vi "Client Test.vi"() -> ()   [LabVIEW 2019, in "Simple_client.lvlib" / "Simple_client.lvclass"]
uses:
  Simple_client.lvclass
  RPC Messages/simpleMsgReq/simpleMsgReq_Data.ctl
  RPC Messages/simpleMgsReply/simpleMgsReply_Data.ctl
panel:
  out "Response Data":T1
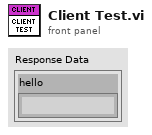
[diagram p1: front panel]
types:
  T1 = typedef "Simple_client.lvlib/Simple_client.lvclass/simpleMgsReply_Data.ctl" = cluster{"hello":string}
  T2 = typedef "Simple_client.lvlib/Simple_client.lvclass/simpleMsgReq_Data.ctl" = cluster{"name":string}
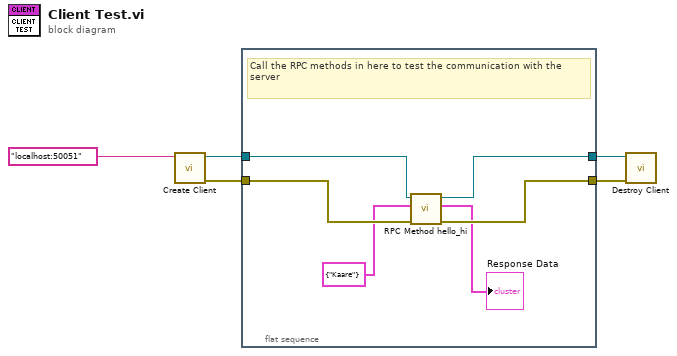
[diagram p0: block diagram]
diagram:
  n1 = call "Create Client.vi"("address"="localhost:50051") -> ("error out"=w1:errorcluster, "gRPC Client out"=w3:refnum<class "Simple_client.lvclass">)  [unwired: 9 in]
  n2 = flat-sequence {
    tunnel: [w10] -> w4
    tunnel: w3 -> [w11]
    tunnel: [w9] -> w2
    tunnel: w1 -> [w8]
    frame #0 {
      # "Call the RPC methods in here to test the communication with the server"
      n3 = call "RPC Method hello_hi.vi"("error in (no error)"=w8, "Request Data"=T2 {"name"="Kaare"}, "gRPC Client in"=w11) -> ("error out"=w9:errorcluster, "Response Data"=→"Response Data":T1, "gRPC Client out"=w10:refnum<class "Simple_client.lvclass">)  [unwired: 6 in]
    }
  }
  n4 = call "Destroy Client.vi"("error in (no error)"=w2, "gRPC Client in"=w4) -> ()  [unwired: 8 in, 2 out]
